vi "2) Group Publishing.vi"() -> ()   [LabVIEW 2020, in "VectoScratch.lvlib"]
uses:
  VectoScratch.lvlib
  Vecto/Group Info.ctl
  Vecto/Publish Config.ctl
  Vecto/Group Data Type.ctl
  Vecto/Channel Init.ctl
  4d34a514-e5b9-4f11-b735-09902ffeac7b.vi
  Vecto/Group DBL/Group DBL.lvclass
  C:/dev/lv20CE/relink/lv-vecto/Vecto/Group/Group.lvclass
  Vecto/ChannelService/Create Group Abstract.vi
  Vecto/ChannelService/ChannelService.lvclass
  Vecto/RemoteDataService/RemoteDataService.lvclass
  VectoConfig/VectoConfig.lvlib
  Vecto/Group Config/Group Config.lvclass
  Vecto/SequenceCountService/SequenceCountService.lvclass
panel:
  in  "Rate":i32=10
  out "error out":errorcluster
  out "i":i32
  in  "stop":bool
  in  "Publish Address":string="230.0.0.100"
  in  "Publish Port":u16=20000
  in  "Values":dbl[](array[slide])=[0.0, 0.0, 0.0, 0.0, 0.0] scale=0.0..1000.0
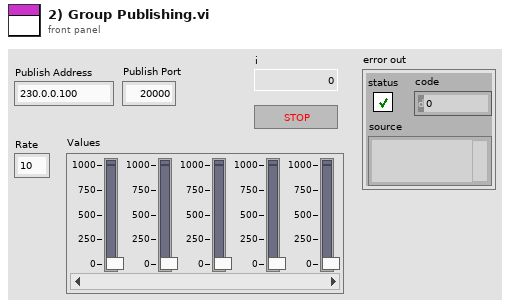
[diagram p1: front panel]
types:
  T1 = typedef "VectoConfig.lvlib/Group Data Type.ctl" = enum16{"Double", "String"}
  T2 = typedef "VectoConfig.lvlib/Publish Config.ctl" = cluster{"Address":string, "Port":u16}
  T3 = typedef "VectoConfig.lvlib/Group Info.ctl" = cluster{"System":string, "Cluster":string, "Node":string, "Task":string, "Name":string}
  T4 = typedef "VectoConfig.lvlib/Channel Init.ctl" = cluster{"Name":string, "Resource":string, "Unit String":string}
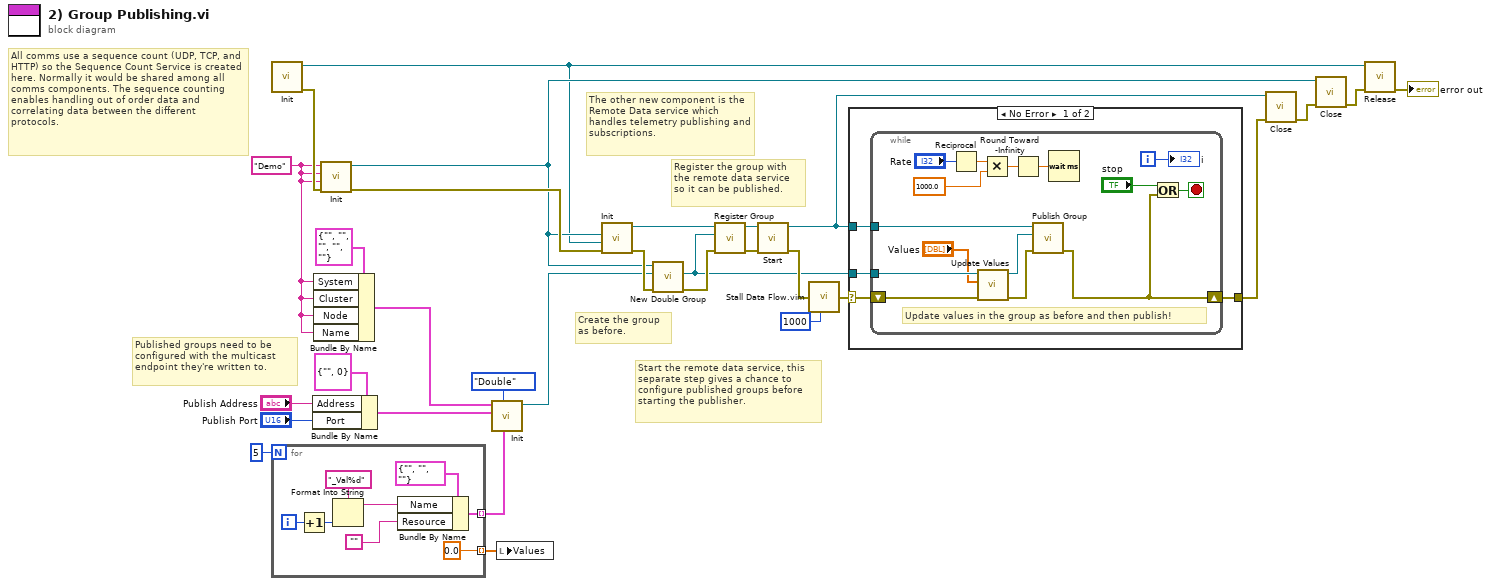
[diagram p0: block diagram]
diagram:
  w4 = "Demo" ("System")
  # "Start the remote data service, this separate step gives a chance to configure published groups before starting the publisher."
  # "Register the group with the remote data service so it can be published."
  # "Create the group as before."
  # "The other new component is the Remote Data service which handles telemetry publishing and subscriptions."
  # "Published groups need to be configured with the multicast endpoint they're written to."
  # "All comms use a sequence count (UDP, TCP, and HTTP) so the Sequence Count Service is created here. Normally it would be shared among all comms components. The sequence counting enables handling out of order data and correlating data between the different protocols."
  n1 = call "Init.vi"() -> ("error out"=w26:errorcluster, "SequenceCountService out"=w11:refnum<class "SequenceCountService.lvclass">)  [unwired: 10 in]
  n2 = for {
    N: 5 -> [_]
    tunnel: [w32] -> w5 mode=indexing
    tunnel: [0.0] -> w2 mode=indexing
    i -> [w38]
    n3 = Increment(x=w38) -> (x+1=w37:i32)
    n4 = Format Into String(format string="_Val%d", w37) -> (resulting string=w35:string)  [unwired: 2 in, 1 out]
    n5 = Bundle By Name(cluster=T4 {"Name"="", "Resource"="", "Unit String"=""} ("Channel Init"), "Name"=w35, "Resource"="") -> (w32:T4)
  }
  n6 = Bundle By Name(cluster=T2 {"Address"="", "Port"=0} ("Publish Config"), "Address"="Publish Address", "Port"="Publish Port") -> (w6:T2)
  n7 = Bundle By Name(cluster=T3 {"System"="", "Cluster"="", "Node"="", "Task"="", "Name"=""} ("Group Info"), "System"=w4, "Cluster"=w4, "Node"=w4, "Name"=w4) -> (w7:T3)
  n8 = call "Init.vi"("error in (no error)"=w26, "Node"=w4, "Cluster"=w4, "System"=w4) -> ("error out"=w27:errorcluster, "ChannelService out"=w13:refnum<class "ChannelService.lvclass">)  [unwired: 6 in]
  n9 = call "Init.vi"("Channels"=w5, "Group Data Type"=Group_Data_Type."Double", "Publish Config (None)"=w6, "Group Info"=w7) -> ("Group Config out"=w23:refnum<class "Group Config.lvclass">)  [unwired: 6 in, 1 out]
  n10 = local write "Values"(w2) -> ()
  n11 = call "Init.vi"("error in (no error)"=w27, "SequenceCountService"=w11, "ChannelService"=w13) -> ("error out"=w29:errorcluster, "RemoteDataService out"=w19:refnum<class "RemoteDataService.lvclass">)  [unwired: 7 in]
  n12 = call "New Double Group.vi"("error in (no error)"=w29, "Group Config"=w23, "ChannelService in"=w13) -> ("error out"=w30:errorcluster, "Group"=w22:refnum<class "Group DBL.lvclass">)  [unwired: 6 in, 1 out]
  n13 = call "Register Group.vi"("error in (no error)"=w30, "Group"=w22, "RemoteDataService in"=w19) -> ("error out"=w18:errorcluster, "RemoteDataService out"=w17:refnum<class "RemoteDataService.lvclass">)  [unwired: 7 in]
  n14 = call "Start.vi"("error in (no error)"=w18, "RemoteDataService in"=w17) -> ("error out"=w28:errorcluster, "RemoteDataService out"=w15:refnum<class "RemoteDataService.lvclass">)  [unwired: 8 in]
  n15 = call "Stall Data Flow.vim"("value in"=w28, "milliseconds to wait"=u32 1000) -> ("value out"=w21:errorcluster)  [unwired: 1 out]
  n16 = case shown="No Error" w21 {
    selector: w21 -> [w40 w58]
    tunnel: [w42 w58] -> w16
    tunnel: w22 -> [w41 _]
    tunnel: w15 -> [w39 _]
    frame No Error {
      n17 = while {
        shift-right: [w57] -> w42
        shift-left: w40 -> [w56]
        tunnel: w41 -> [w54]
        tunnel: w39 -> [w52]
        i -> [w51]
        stop <- w53 stop-if-true
        # "Update values in the group as before and then publish!"
        n18 = Reciprocal(x="Rate") -> (1/x=w49:dbl)
        n19 = call "Update Values.vi"("error in (no error)"=w56, "Values"="Values", "Group in"=w54) -> ("error out"=w43:errorcluster, "Group out"=w44:refnum<class "Group DBL.lvclass">)  [unwired: 7 in]
        n20 = Multiply(x=w49, y=1000.0) -> (x*y=w47:dbl)
        n21 = Round Toward -Infinity(1:w47) -> (0:w46:dbl)
        n22 = call "Publish Group.vi"("error in (no error)"=w43, "Group"=w44, "RemoteDataService in"=w52) -> ("error out"=w57:errorcluster)  [unwired: 7 in, 1 out]
        n23 = Wait (ms)(milliseconds to wait=w46) -> ()  [unwired: 1 out]
        n24 = Or(x="stop", y=w57) -> (x .or. y?=w53:bool)
        "i" <- w51
      }
    }
    frame Error {
    }
  }
  n25 = call "Close.vi"("error in (no error)"=w16, "RemoteDataService in"=w15) -> ("error out"=w14:errorcluster)  [unwired: 9 in]
  n26 = call "Close.vi"("error in (no error)"=w14, "ChannelService in"=w13) -> ("error out"=w12:errorcluster)  [unwired: 9 in]
  n27 = call "Release.vi"("error in (no error)"=w12, "SequenceCountService in"=w11) -> ("error out"=→"error out":errorcluster)  [unwired: 9 in]
